vi "Scope_Init.vi"(8 "Error In":errorcluster, 10 "HW Device Name":string, 11 "Object in":refnum<class "Scope.lvclass">) -> (0 "Error Out":errorcluster, 3 "object out":refnum<class "Scope.lvclass">)   [LabVIEW 2023, in "HAL.lvlib" / "Scope.lvclass"]
uses:
  Scope.lvclass
  Scope.lvclass/Scope.ctl
  Hardware_class/Hardware.lvclass
  D:/git/HAL/Hardware_class/Hardware.lvclass
  D:/git/HAL/Scope_class/Scope.lvclass
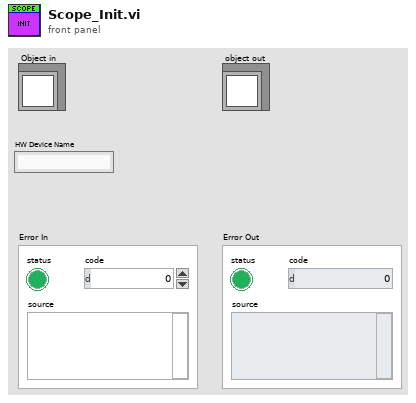
[diagram p1: front panel]
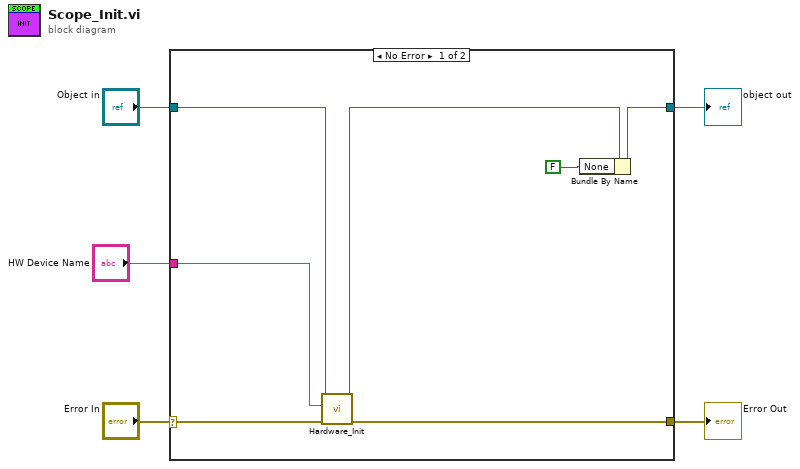
[diagram p0: block diagram]
diagram:
  n1 = case shown="No Error" "Error In" {
    selector: "Error In" -> [w10 w13]
    tunnel: [w12 w14] -> w5
    tunnel: "Object in" -> [w8 w14]
    tunnel: [w9 w13] -> w2
    tunnel: "HW Device Name" -> [w6 _]
    frame No Error {
      n2 = call "Hardware_Init.vi"("Error In"=w10, "HW Device Name"=w6, "object in"=w8) -> ("Error Out"=w9:errorcluster, "object out"=w7:refnum<class "Scope.lvclass">)  [unwired: 7 in]
      n3 = Bundle By Name(cluster=w7, "None"=FALSE) -> (w12:refnum<class "Scope.lvclass">)
    }
    frame Error {
    }
  }
  "object out" <- w5
  "Error Out" <- w2
